vi "FTW-ActorExtended-Children-PoisonPill.vi"(0 "FTW-ActorExtended In":refnum<class "FTW-ActorExtended.lvclass">, 9 "Timeout":i32=100 format="%dmsec", 11 "error in":errorcluster) -> (4 "FTW-ActorExtended Out":refnum<class "FTW-ActorExtended.lvclass">, 15 "error out":errorcluster)   [LabVIEW 2015, in "FTW-ActorExtended.lvclass"]
uses:
  FTW-ActorExtended.lvclass
  FTW-ActorExtended.lvclass/FTW-ActorExtended.ctl
  Connector/FTW-ActorConnector.lvclass
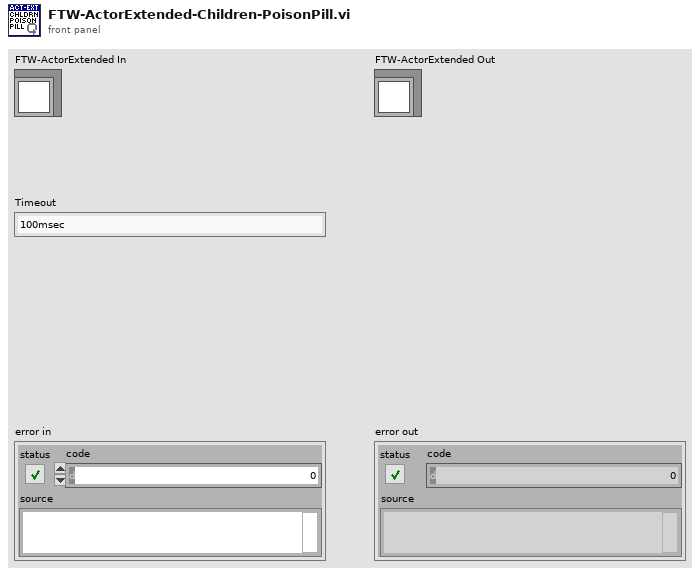
[diagram p1: front panel]
types:
  T1 = cluster{"Name":string, "URI":string, "Connector":refnum<class "FTW-ActorConnector.lvclass">, "Child":bool}[]
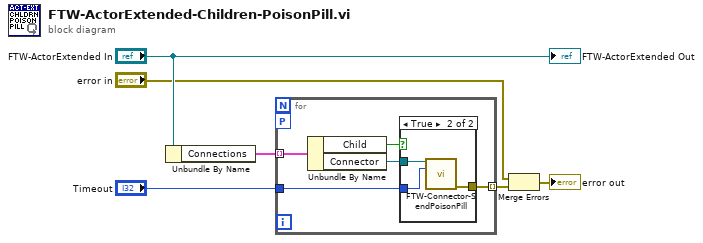
[diagram p0: block diagram]
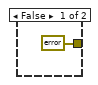
[diagram p2: hidden frame]
diagram:
  n1 = Unbundle By Name("FTW-ActorExtended In") -> ("Connections"=w3:T1)
  n2 = for {
    tunnel: [w11] -> w5 mode=indexing
    tunnel: "Timeout" -> [w10]
    tunnel: w3 -> [w8] mode=indexing
    workers-P: _ -> [_]
    n3 = Unbundle By Name(w8) -> ("Child"=w7:bool, "Connector"=w9:refnum<class "FTW-ActorConnector.lvclass">)
    n4 = case shown="True" w7 {
      tunnel: [errorcluster {"status"=FALSE, "code"=0, "source"=""} ("error out") w15] -> w11
      tunnel: w10 -> [_ w14]
      tunnel: w9 -> [_ w13]
      frame False {
      }
      frame True {
        n5 = call-dynamic "FTW-Connector-SendPoisonPill.vi"("FTW Actor Connector"=w13, "Timeout"=w14) -> ("error out"=w15:errorcluster)  [unwired: 8 in, 5 out]
      }
    }
  }
  n6 = Merge Errors("error in", w5) -> (→"error out":errorcluster)
  "FTW-ActorExtended Out" <- "FTW-ActorExtended In"
